vi "0xE9_Read_description_one_telem_parameter.vi"(8 "error in (no error)":errorcluster, 10 "NumberTelemParam":i32 format="%0d", 11 "paramUnicornIn in":T2) -> (0 "error out":errorcluster, 1 "Param":T1, 3 "paramUnicornIn out 2":T2)   [LabVIEW 2017, in "LV_Unicorn.lvlib"]
uses:
  LV_Unicorn.lvlib
  Control/unicorn_Param.ctl
  Control/unicorn_conn.ctl
  Control/unicorn_JSON.ctl
  Control/unicorn_ParamInt.ctl
  Control/unicorn_Telemetry.ctl
  Control/unicorn_Table.ctl
  Control/unicorn_ParamFloat.ctl
  Control/unicorn_DescriptParam.ctl
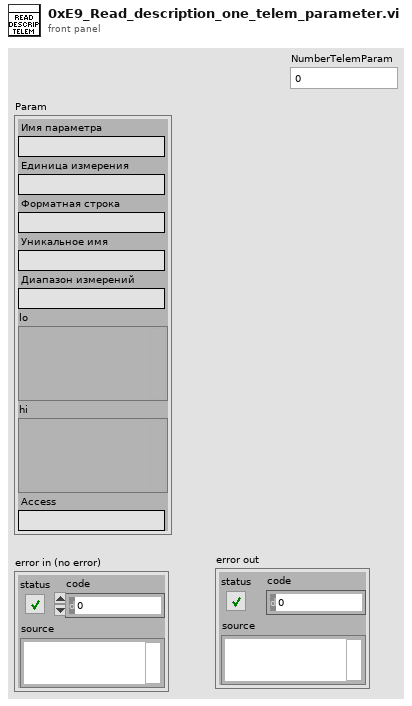
[diagram p1: front panel]
types:
  T1 = typedef "unicorn_DescriptParam.ctl" = cluster{"Имя параметра":string, "Единица измерения":string, "Форматная строка ":string, "Уникальное имя":string, "Диапазон измерений":string, "lo":variant, "hi":variant, "Access":string}
  T2 = typedef "LV_Unicorn.lvlib/unicorn_Param.ctl" = cluster{"conParam":T3, "Param":T4}
  T3 = typedef "LV_Unicorn.lvlib/unicorn_conn.ctl" = cluster{"ReadIntParam":bool, "ReadDescrParam":bool, "ReadFloatParam":bool, "debug":bool, "ReadJSON":bool, "IP_address":string, "N_attempts":i32, "type_con":enum16{"Serial", "TCP"}, "MB_address":i32, "VISA":refnum<visa-resource-name>, "connection ID":refnum<k5>, "nameDevices":string, "timeout":i32, "port":u16, "type_version":string, "baud_rate":u32, "VersionControl":bool, "TCP_conn":bool, "WindowSize":i32}
  T4 = typedef "LV_Unicorn.lvlib/unicorn_JSON.ctl" = cluster{"NumParam":cluster{"NTelem":i32, "NInt":i32, "NFloat":i32, "NTable":i32}, "ParamInt":T5, "Telemetry":T6, "Table":T7, "ParamFloat":T8}
  T5 = typedef "LV_Unicorn.lvlib/unicorn_ParamInt.ctl" = cluster{"ID":string, "Num":i32, "Name":string, "Type":string, "Enum":string, "Desc":string, "Unit":string, "Access":string, "FormatStr":string, "Min":i32, "Max":i32}[]
  T6 = typedef "LV_Unicorn.lvlib/unicorn_Telemetry.ctl" = cluster{"ID":string, "Num":i32, "Name":string, "Desc":string, "Unit":string, "FormatStr":string, "Min":i32, "Max":i32}[]
  T7 = typedef "LV_Unicorn.lvlib/unicorn_Table.ctl" = cluster{"Num":i32, "Access":string, "ColumnCount":i32, "NeedParamPrepare":bool, "Columns":cluster{"Column":i32, "Desc":string, "Name":string}[], "DataType":string, "FormatStr":string, "ID":string, "Name":string, "RowCount":i32, "Rows":cluster{"Desc":string, "ID":string, "Max":i32, "Min":i32, "Name":string, "Row":i32, "Unit":string}[], "Type":string}[]
  T8 = typedef "LV_Unicorn.lvlib/unicorn_ParamFloat.ctl" = cluster{"ID":string, "Num":i32, "Name":string, "Type":string, "Enum":string, "Desc":string, "Unit":string, "Access":string, "FormatStr":string, "Min":sgl, "Max":sgl}[]
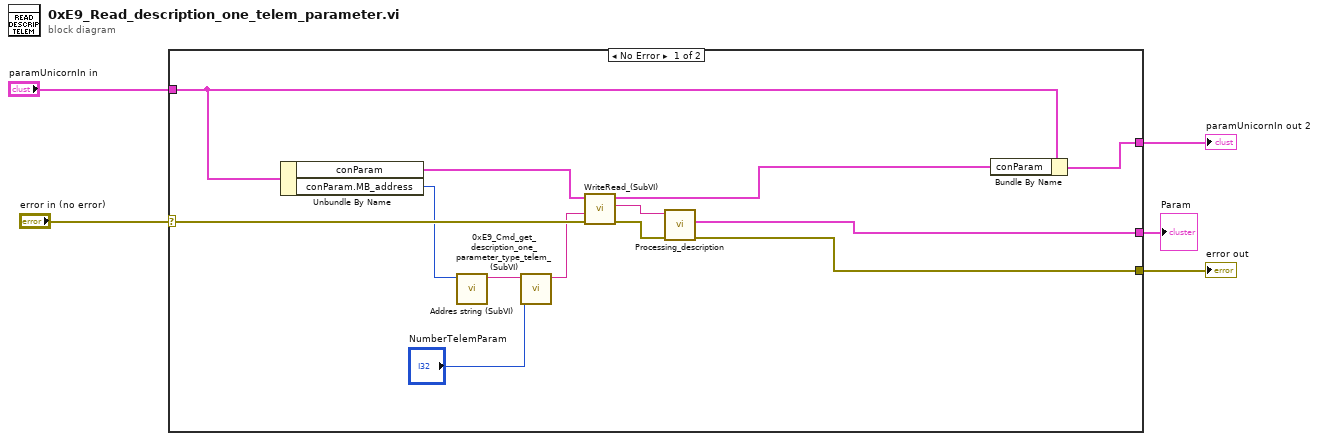
[diagram p0: block diagram]
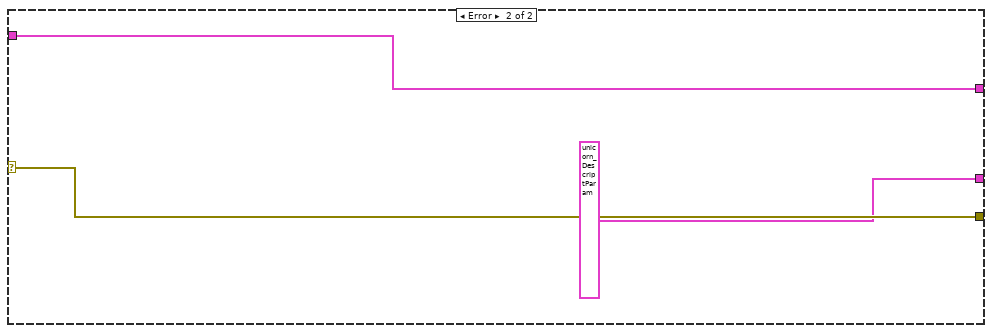
[diagram p2: hidden frame]
diagram:
  n1 = case shown="No Error" "error in (no error)" {
    selector: "error in (no error)" -> [w17 w21]
    tunnel: [w14 w21] -> w5
    tunnel: "paramUnicornIn in" -> [w10 w20]
    tunnel: [w12 w20] -> w3
    tunnel: [w13 T1 {"Имя параметра"="", "Единица измерения"="", "Форматная строка "="", "Уникальное имя"="", "Диапазон измерений"="", "lo"=variant, "hi"=variant, "Access"=""} ("Param")] -> w1
    frame No Error {
      n2 = Unbundle By Name(w10) -> ("conParam"=w18:T3, "conParam.MB_address"=w9:i32)
      n3 = call "Addres string (SubVI).vi"("Адрес"=w9) -> ("String"=w8:string)  [unwired: 10 in]
      n4 = call "0xE9_Cmd_get_description_one_parameter_type_telem_(SubVI).vi"("NumberTelemParam"="NumberTelemParam", "String in"=w8) -> ("String out"=w7:string)  [unwired: 9 in]
      n5 = call "WriteRead_(SubVI).vi"("error in"=w17, "Запрос"=w7, "ParamIn"=w18) -> ("error out"=w16:errorcluster, "Ответ"=w15:string, "ParamOut"=w11:T3)  [unwired: 4 in, 2 out]
      n6 = call "Processing_description.vi"("error in"=w16, "Ответ устройства"=w15) -> ("error out"=w14:errorcluster, "Param"=w13:T1)  [unwired: 6 in, 2 out]
      n7 = Bundle By Name(cluster=w10, "conParam"=w11) -> (w12:T2)
    }
    frame Error {
    }
  }
  "error out" <- w5
  "paramUnicornIn out 2" <- w3
  "Param" <- w1
